vi "manejaBD.vi"(8 "error in":errorcluster, 10 "All Message Queues in":T1, 11 "Sonometro in":refnum<class "Sonometro.lvclass">) -> (0 "error out":errorcluster)   [LabVIEW 2019, in "Sonometro.lvclass"]
uses:
  Sonometro.lvclass
  QMH/Message Queue/All Message Queues.ctl
  QMH/Message Queue/Message Cluster.ctl
  Sonometro.lvclass/Sonometro.ctl
  <vilib>/Utility/error.llb/Error Cluster From Error Code.vi
  RerenceAllControlsToolkit/_get mutiple control reference by name.vi
  RerenceAllControlsToolkit/_get control reference by name.vi
  QMH/Message Queue/Enqueue Message (Single).vi
  <vilib>/ErrorRing/Error Ring.xnode
  Base de Datos/SQLiteConnector/SQLiteConnection.lvclass
  QMH/Message Queue/Message Queue.lvlib
  Base de Datos/Base de Datos.lvclass
  <vilib>/Utility/Data Type/NI_Data Type.lvlib
panel:
  out "All States":string[](array[string])
  out "Actual State":string
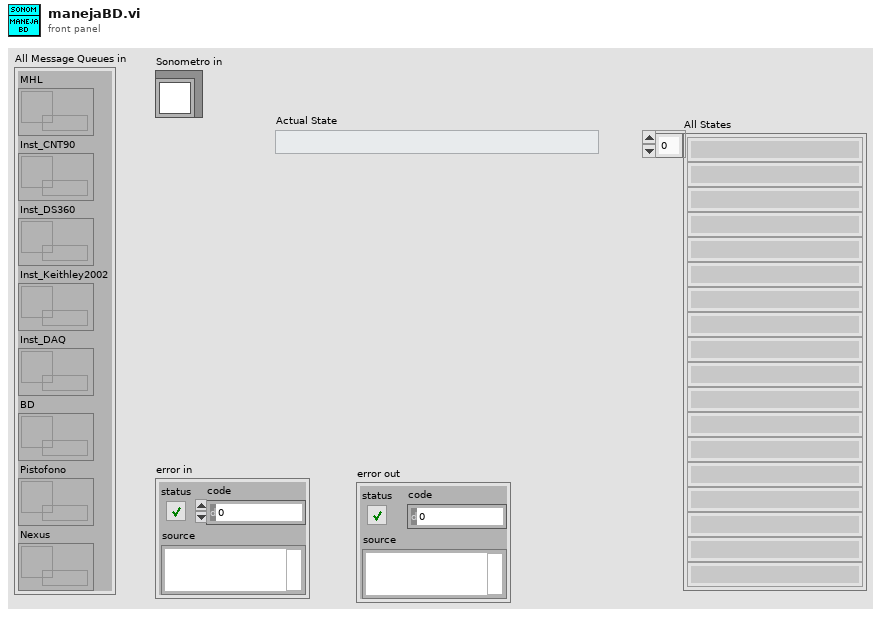
[diagram p1: front panel]
types:
  T1 = typedef "Message Queue.lvlib/All Message Queues.ctl" = cluster{"MHL":refnum<queue>, "Inst_CNT90":refnum<queue>, "Inst_DS360":refnum<queue>, "Inst_Keithley2002":refnum<queue>, "Inst_DAQ":refnum<queue>, "BD":refnum<queue>, "Pistofono":refnum<queue>, "Nexus":refnum<queue>}
  T2 = cluster{"Marca":string, "Referencia":cluster{"ControlName":string, "ControlReference":refnum<vi>}[]}
  T3 = typedef "NI_Data Type.lvlib/Data Type.ctl" = enum8{"Invalid Type", "Void", "I8", "I16", "I32", "I64", "U8", "U16", "U32", "U64", "Single Float", "Double Float", "Extended Float", "Single Complex", "Double Complex", "Extended Complex", "Enum U8", "Enum U16", "Enum U32", "Enum U64", "Single Float With Unit", "Double Float With Unit", "Extended Float With Unit", "Single Complex with Unit", "Double Complex with Unit", "Extended Complex with Unit", "Boolean", "String", "Path", "Picture", "Tag", "Array", "Cluster", "Variant", "LV Variant", "Waveform", "Timestamp", "Digital Waveform", "Digital Data", "ExpressData", "Refnum", "External Data", "VI", "Poly VI", "LabVIEW Class Instance", "Fixed Point", "Set Collection", "Map Collection"}
  T4 = cluster{"ControlName":string, "ControlReference":refnum<vi>}[]
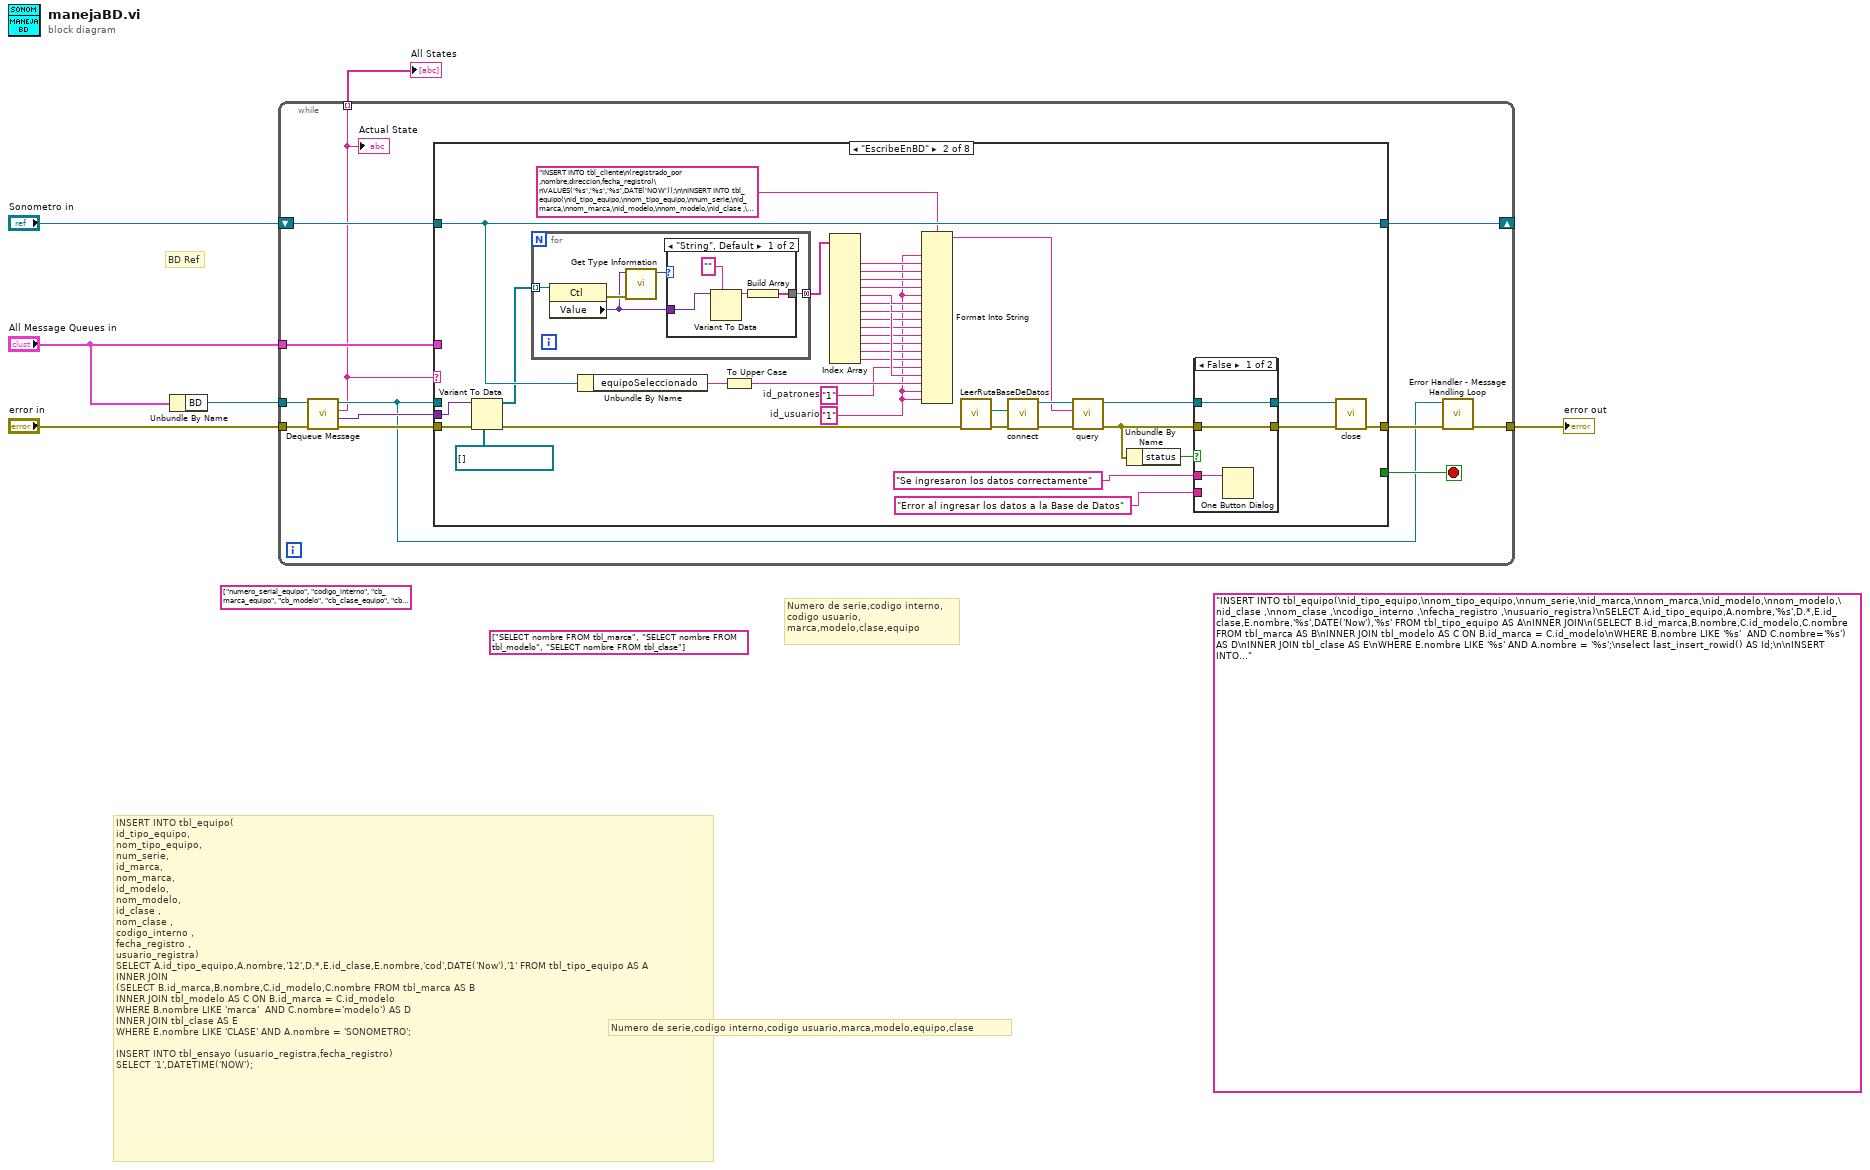
[diagram p0: block diagram]
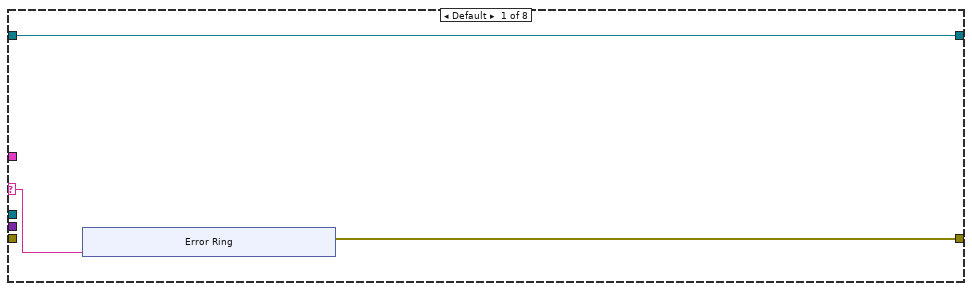
[diagram p2: hidden frame]
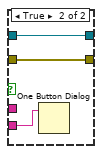
[diagram p3: hidden frame]
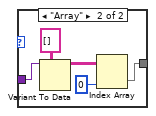
[diagram p4: hidden frame]
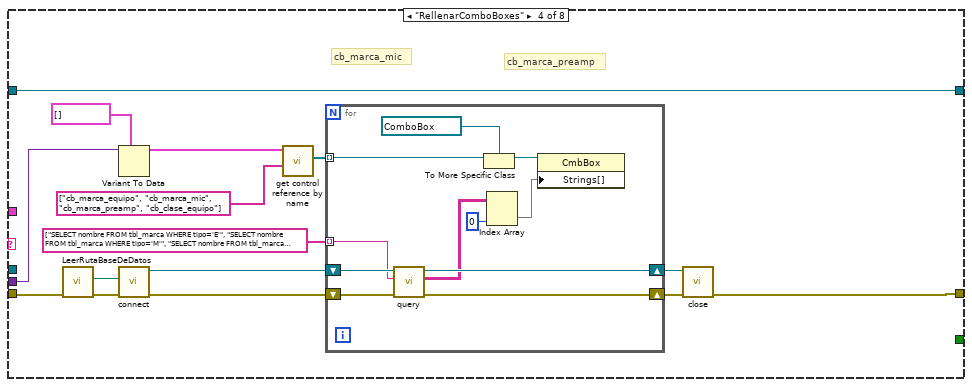
[diagram p6: hidden frame]
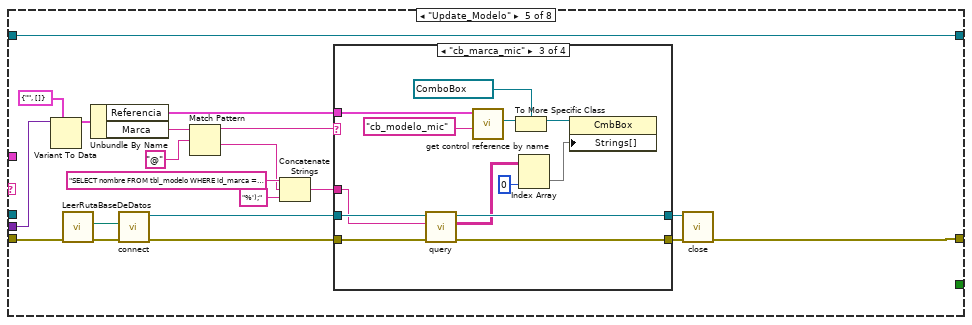
[diagram p7: hidden frame]
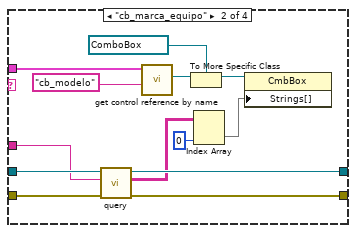
[diagram p9: hidden frame]
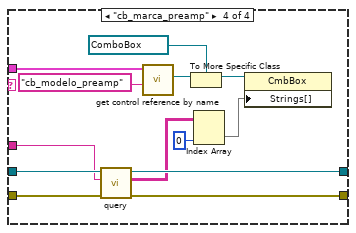
[diagram p10: hidden frame]
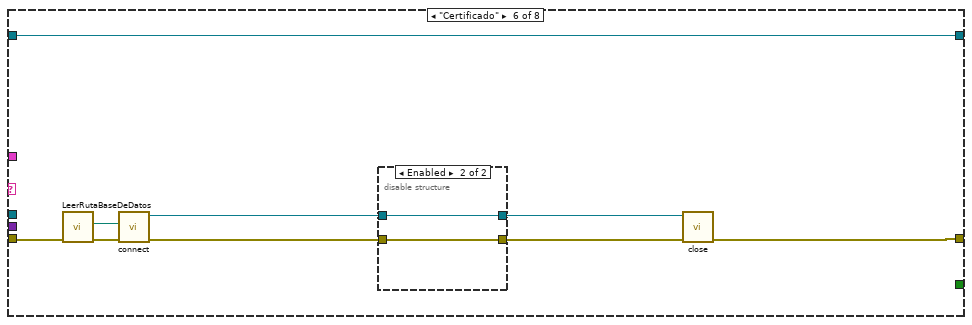
[diagram p11: hidden frame]
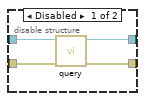
[diagram p12: hidden frame]
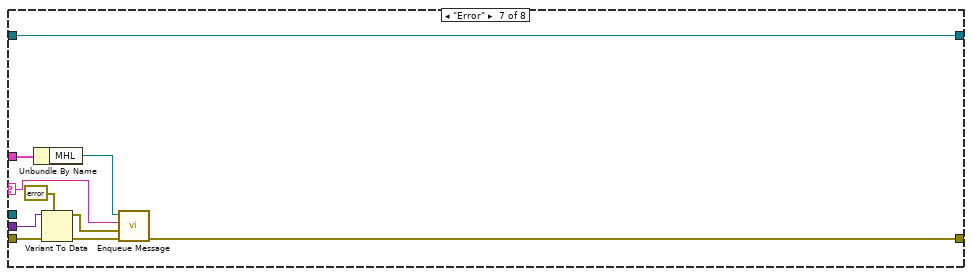
[diagram p13: hidden frame]
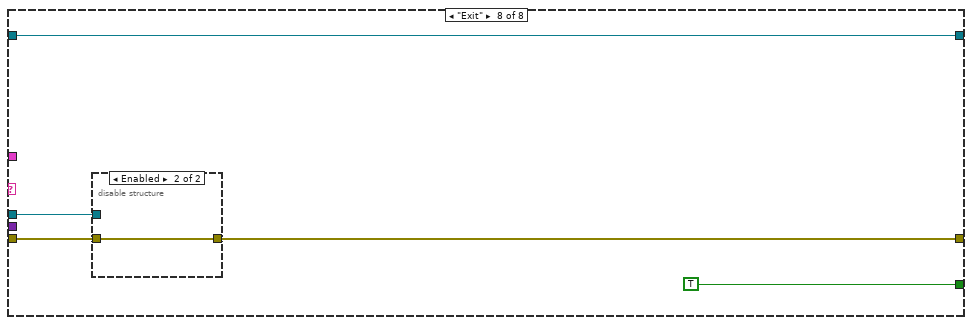
[diagram p14: hidden frame]
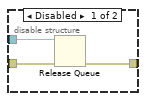
[diagram p15: hidden frame]
diagram:
  (unwired) string[] ["numero_serial_equipo", "codigo_interno", "cb_marca_equipo", "cb_modelo", "cb_clase_equipo", "cb_marca_mic", "cb_modelo_mic", "numero_serial_mic", "cb_marca_preamp", "cb_modelo_preamp", "numero_serial_preamp"]
  (unwired) "INSERT INTO tbl_equipo(\nid_tipo_equipo,\nnom_tipo_equipo,\nnum_serie,\nid_marca,\nnom_marca,\nid_modelo,\nnom_modelo,\nid_clase ,\nnom_clase ,\ncodigo_interno ,\nfecha_registro ,\nusuario_registra)\nSELECT A.id_tipo_equipo,A.nombre,'%s',D.*,E.id_clase,E.nombre,'%s',DATE('Now'),'%s' FROM tbl_tipo_equipo AS A\nINNER JOIN\n(SELECT B.id_marca,B.nombre,C.id_modelo,C.nombre FROM tbl_marca AS B\nINNER JOIN tbl_modelo AS C ON B.id_marca = C.id_modelo\nWHERE B.nombre LIKE '%s'  AND C.nombre='%s') AS D\nINNER JOIN tbl_clase AS E\nWHERE E.nombre LIKE '%s' AND A.nombre = '%s';\nselect last_insert_rowid() AS Id;\n\nINSERT INTO tbl_info_ensayo (id_ensayo,id_equipo,id_cliente,id_cond_amb_iniciales,id_clase_pruebas)\nSELECT (SELECT MAX(id_ensayo) FROM tbl_ensayo) AS id_ensayo,(SELECT MAX(id_equipo) FROM tbl_equipo) AS id_equipo,'%s' AS id_cliente,(SELECT MAX(id_cond_amb_iniciales) FROM tbl_cond_amb_iniciales) AS id_cond_amb_iniciales,\n(SELECT id_clase_prueba FROM tbl_clase_prueba WHERE id_clase=(SELECT id_clase FROM tbl_equipo ORDER BY id_equipo DESC LIMIT 1)  AND id_prueba=(SELECT id_prueba FROM tbl_prueba Where nombre='%s')) AS id_clase_pruebas;\n"
  (unwired) string[] ["SELECT nombre FROM tbl_marca", "SELECT nombre FROM tbl_modelo", "SELECT nombre FROM tbl_clase"]
  # "INSERT INTO tbl_equipo(\nid_tipo_equipo,\nnom_tipo_equipo,\nnum_serie,\nid_marca,\nnom_marca,\nid_modelo,\nnom_modelo,\nid_clase ,\nnom_clase ,\ncodigo_interno ,\nfecha_registro ,\nusuario_registra)\nSELECT A.id_tipo_equipo,A.nombre,'12',D.*,E.id_clase,E.nombre,'cod',DATE('Now'),'1' FROM tbl_tipo_equipo AS A\nINNER JOIN\n(SELECT B.id_marca,B.nombre,C.id_modelo,C.nombre FROM tbl_marca AS B\nINNER JOIN tbl_modelo AS C ON B.id_marca = C.id_modelo\nWHERE B.nombre LIKE 'marca'  AND C.nombre='modelo') AS D\nINNER JOIN tbl_clase AS E\nWHERE E.nombre LIKE 'CLASE' AND A.nombre = 'SONOMETRO';\n\nINSERT INTO tbl_ensayo (usuario_registra,fecha_registro)\nSELECT '1',DATETIME('NOW');"
  # "Numero de serie,codigo interno,\ncodigo usuario,\nmarca,modelo,clase,equipo"
  # "Numero de serie,codigo interno,codigo usuario,marca,modelo,equipo,clase"
  # "BD Ref"
  n1 = Unbundle By Name("All Message Queues in") -> ("BD"=w4:refnum<queue>)
  n2 = while {
    tunnel: "error in" -> [w18]
    tunnel: w4 -> [w17]
    tunnel: "All Message Queues in" -> [w16]
    tunnel: [w9] -> w2
    shift-right: [w12] -> _
    shift-left: "Sonometro in" -> [w15]
    tunnel: [w7] -> w1 mode=indexing
    stop <- w11 stop-if-true
    n3 = call "Dequeue Message.vi"("error in (no error)"=w18, "Message Queue"=w17) -> ("error out"=w13:errorcluster, "Message Data"=w14:variant, "Message"=w7:string, "dup Message Queue"=w8:refnum<queue>)  [unwired: 6 in]
    "Actual State" <- w7
    n4 = case shown="\"EscribeEnBD\"" w7 {
      selector: w7 -> [w21 _ _ _ _ _ w195 _]
      tunnel: w16 -> [_ _ _ _ _ _ w194 _]
      tunnel: w15 -> [w19 w61 w88 w89 w134 w184 w192 w202]
      tunnel: w8 -> [_ _ _ _ _ _ _ w204]
      tunnel: w14 -> [_ w63 _ w96 w126 _ w198 _]
      tunnel: w13 -> [_ w65 w87 w99 w129 w179 w199 w205]
      tunnel: [w20 w66 w87 w97 w127 w177 w191 w201] -> w10
      tunnel: [w19 w61 w88 w89 w134 w184 w192 w202] -> w12
      tunnel: [_ _ _ _ _ _ _ TRUE] -> w11
      frame Default {
        n5 = xnode "Error Ring"("parameter 0"=w21) -> ("error out"=w20:errorcluster)
      }
      frame "EscribeEnBD" {
        w47 = "1"  # id_patrones
        w36 = "1"  # id_usuario
        n6 = Variant To Data(error in=w65, type=refnum<vi>[] [], Variant=w63) -> (data=w40:refnum<vi>[], error out=w64:errorcluster)
        n7 = for {
          tunnel: w40 -> [w77] mode=indexing
          tunnel: [w76] -> w39 mode=concatenating
          n8 = property class="Ctl"(reference=w77) -> (error out=w75:errorcluster, "Value"=w74:variant)  [unwired: 1 in, 1 out]
          n9 = call <vilib>:"Get Type Information.vi"("error in (no error)"=w75, "variant"=w74) -> ("type"=w73:T3)  [unwired: 5 in, 4 out]
          n10 = case shown="\"String\", Default" w73 {
            tunnel: [w78 w83] -> w76
            tunnel: w74 -> [w80 w85]
            frame "String", Default {
              n11 = Variant To Data(type="", Variant=w80) -> (data=w79:string)  [unwired: 1 in, 1 out]
              n12 = Build Array(w79) -> (w78:string[])
            }
            frame "Array" {
              n13 = Variant To Data(type=string[][] [], Variant=w85) -> (data=w84:string[][])  [unwired: 1 in, 1 out]
              n14 = Index Array(array=w84, index (col)=0 ("disabled index (col)")) -> (element=w83:string[])  [unwired: 1 in]
            }
          }
        }
        n15 = Unbundle By Name(w61) -> ("equipoSeleccionado"=w50:string)
        n16 = To Upper Case(1:w50) -> (0:w49:string)
        n17 = Index Array(array=w39) -> (element #2=w37:string, element #3=w38:string, element #4=w55:string, element #5=w54:string, element #6=w53:string, element #7=w52:string, element #8=w48:string, element #9=w46:string, element #10=w45:string, element #11=w44:string, element #12=w43:string, element #13=w42:string, element #14=w41:string)  [unwired: 14 in, 1 out]
        n18 = Format Into String(format string="INSERT INTO tbl_cliente\n(registrado_por ,nombre,direccion,fecha_registro)\nVALUES('%s','%s','%s',DATE('NOW'));\n\nINSERT INTO tbl_equipo(\nid_tipo_equipo,\nnom_tipo_equipo,\nnum_serie,\nid_marca,\nnom_marca,\nid_modelo,\nnom_modelo,\nid_clase ,\nnom_clase ,\ncodigo_interno ,\nfecha_registro ,\nusuario_registra,\nmarca_microfono,\nmodelo_microfono,\nnum_serie_microfono,\nmarca_preamplificador ,\nmodelo_preamplificador,\nnum_serie_preamplificador,\nid_patrones_calib)\nSELECT A.id_tipo_equipo,A.nombre,'%s',D.*,E.id_clase,E.nombre,'%s',DATE('Now'),'%s',F.* FROM tbl_tipo_equipo AS A\nINNER JOIN\n(SELECT B.id_marca,B.nombre,C.id_modelo,C.nombre FROM tbl_marca AS B\nINNER JOIN tbl_modelo AS C ON B.id_marca = C.id_marca\nWHERE B.nombre LIKE '%s'  AND C.nombre='%s') AS D\nINNER JOIN tbl_clase AS E\nINNER JOIN (SELECT '%s','%s','%s','%s','%s','%s','%s') AS F\nWHERE E.nombre LIKE '%s' AND A.nombre = '%s';\n\nINSERT INTO tbl_equipo_cliente(id_cliente,nom_cliente,id_equipo,fecha_registro,usuario_registra)\nSELECT MAX(id_cliente),nombre,last_insert_rowid(),DATETIME('NOW'),'%s' FROM tbl_cliente;\n\nINSERT INTO tbl_ensayo (usuario_registra,fecha_registro)\nSELECT '%s',DATETIME('NOW');\n", w36, w37, w38, w55, w54, w36, w53, w52, w46, w45, w44, w43, w42, w41, w47, w48, w49, w36, w36) -> (resulting string=w51:string)  [unwired: 2 in, 1 out]
        n19 = call "LeerRutaBaseDeDatos.vi"("error in (no error)"=w64) -> ("error out"=w58:errorcluster, "Database Path"=w57:path)  [unwired: 9 in]
        n20 = call "connect.vi"("error in (no error)"=w58, "Database Path"=w57) -> ("error out"=w60:errorcluster, "object out"=w59:refnum<class "SQLiteConnection.lvclass">)  [unwired: 8 in]
        n21 = call "query.vi"("error in (no error)"=w60, "SQL Statement"=w51, "object in"=w59) -> ("error out"=w32:errorcluster, "object out"=w34:refnum<class "SQLiteConnection.lvclass">)  [unwired: 5 in, 2 out]
        n22 = Unbundle By Name(w32) -> ("status"=w35:bool)
        n23 = case shown="False" w35 {
          tunnel: w34 -> [w69 w72]
          tunnel: [w69 w72] -> w33
          tunnel: w32 -> [w68 w71]
          tunnel: [w68 w71] -> w31
          tunnel: "Se ingresaron los datos correctamente" -> [w67 _]
          tunnel: "Error al ingresar los datos a la Base de Datos" -> [_ w70]
          frame False {
            n24 = One Button Dialog(message=w67) -> ()  [unwired: 1 in, 1 out]
          }
          frame True {
            n25 = One Button Dialog(message=w70) -> ()  [unwired: 1 in, 1 out]
          }
        }
        n26 = call-dynamic "close.vi"("error in (no error)"=w31, "object in"=w33) -> ("error out"=w66:errorcluster)  [unwired: 8 in, 1 out]
      }
      frame "Initialize" {
      }
      frame "RellenarComboBoxes" {
        # "cb_marca_preamp"
        # "cb_marca_mic"
        n27 = call "LeerRutaBaseDeDatos.vi"("error in (no error)"=w99) -> ("error out"=w101:errorcluster, "Database Path"=w100:path)  [unwired: 9 in]
        n28 = Variant To Data(type=cluster{string, refnum<vi>}[] [] ("Control references"), Variant=w96) -> (data=w94:cluster{string, refnum<vi>}[])  [unwired: 1 in, 1 out]
        n29 = call "connect.vi"("error in (no error)"=w101, "Database Path"=w100) -> ("error out"=w102:errorcluster, "object out"=w103:refnum<class "SQLiteConnection.lvclass">)  [unwired: 8 in]
        n30 = call-poly "get control reference by name.vi"("Control names"=string[] ["cb_marca_equipo", "cb_marca_mic", "cb_marca_preamp", "cb_clase_equipo"] ("Control name"), "Control references"=w94) -> ("References"=w92:refnum<vi>[])  [unwired: 4 in, 1 out]
        n31 = for {
          tunnel: w92 -> [w109] mode=indexing
          shift-right: [w112] -> w98
          shift-left: w103 -> [w114]
          shift-right: [w105] -> w91
          shift-left: w102 -> [w113]
          tunnel: string[] ["SELECT nombre FROM tbl_marca WHERE tipo='E'", "SELECT nombre FROM tbl_marca WHERE tipo='M'", "SELECT nombre FROM tbl_marca WHERE tipo='P'", "SELECT nombre FROM tbl_clase"] -> [w104] mode=indexing
          n32 = call "query.vi"("error in (no error)"=w113, "SQL Statement"=w104, "object in"=w114) -> ("error out"=w105:errorcluster, "result"=w111:string[][], "object out"=w112:refnum<class "SQLiteConnection.lvclass">)  [unwired: 5 in, 1 out]
          n33 = To More Specific Class(target class=refnum<vi> refnum ("cb_marca_equipo"), reference=w109) -> (specific class reference=w108:refnum<vi>)  [unwired: 1 in, 1 out]
          n34 = Index Array(array=w111, index (col)=0 ("disabled index (col)")) -> (element=w106:string[])  [unwired: 1 in]
          n35 = property class="CmbBox"(reference=w108, "Strings[]"=w106) -> ()  [unwired: 1 in, 2 out]
        }
        n36 = call-dynamic "close.vi"("error in (no error)"=w91, "object in"=w98) -> ("error out"=w97:errorcluster)  [unwired: 8 in, 1 out]
      }
      frame "Update_Modelo" {
        n37 = Variant To Data(type=T2 {"Marca"="", "Referencia"=[]} ("output cluster"), Variant=w126) -> (data=w123:T2)  [unwired: 1 in, 1 out]
        n38 = call "LeerRutaBaseDeDatos.vi"("error in (no error)"=w129) -> ("error out"=w131:errorcluster, "Database Path"=w130:path)  [unwired: 9 in]
        n39 = Unbundle By Name(w123) -> ("Referencia"=w122:T4, "Marca"=w120:string)
        n40 = call "connect.vi"("error in (no error)"=w131, "Database Path"=w130) -> ("error out"=w132:errorcluster, "object out"=w133:refnum<class "SQLiteConnection.lvclass">)  [unwired: 8 in]
        n41 = Match Pattern(string=w120, regular expression="@") -> (before substring=w121:string, after substring=w117:string)  [unwired: 1 in, 2 out]
        n42 = Concatenate Strings("SELECT nombre FROM tbl_modelo WHERE id_marca = (SELECT id_marca FROM tbl_marca WHERE nombre LIKE '%" ("SQL Statement"), w117, "%');" ("string")) -> (w115:string)
        n43 = case shown="\"cb_marca_mic\"" w121 {
          tunnel: w133 -> [w136 w149 w162 w175]
          tunnel: w132 -> [w135 w148 w161 w174]
          tunnel: [w136 w147 w160 w173] -> w128
          tunnel: [w135 w145 w158 w171] -> w125
          tunnel: w122 -> [_ w138 w151 w164]
          tunnel: w115 -> [_ w137 w150 w163]
          frame "False", Default {
          }
          frame "cb_marca_equipo" {
            n44 = call "query.vi"("error in (no error)"=w148, "SQL Statement"=w137, "object in"=w149) -> ("error out"=w145:errorcluster, "result"=w144:string[][], "object out"=w147:refnum<class "SQLiteConnection.lvclass">)  [unwired: 5 in, 1 out]
            n45 = call-poly "get control reference by name.vi"("Control name"="cb_modelo", "Control references"=w138) -> ("Ctl Refnum"=w146:refnum<vi>)  [unwired: 4 in, 1 out]
            n46 = To More Specific Class(target class=refnum<vi> refnum ("cb_marca_equipo"), reference=w146) -> (specific class reference=w142:refnum<vi>)  [unwired: 1 in, 1 out]
            n47 = Index Array(array=w144, index (col)=0 ("disabled index (col)")) -> (element=w140:string[])  [unwired: 1 in]
            n48 = property class="CmbBox"(reference=w142, "Strings[]"=w140) -> ()  [unwired: 1 in, 2 out]
          }
          frame "cb_marca_mic" {
            n49 = call "query.vi"("error in (no error)"=w161, "SQL Statement"=w150, "object in"=w162) -> ("error out"=w158:errorcluster, "result"=w157:string[][], "object out"=w160:refnum<class "SQLiteConnection.lvclass">)  [unwired: 5 in, 1 out]
            n50 = call-poly "get control reference by name.vi"("Control name"="cb_modelo_mic", "Control references"=w151) -> ("Ctl Refnum"=w159:refnum<vi>)  [unwired: 4 in, 1 out]
            n51 = To More Specific Class(target class=refnum<vi> refnum ("cb_marca_equipo"), reference=w159) -> (specific class reference=w155:refnum<vi>)  [unwired: 1 in, 1 out]
            n52 = Index Array(array=w157, index (col)=0 ("disabled index (col)")) -> (element=w153:string[])  [unwired: 1 in]
            n53 = property class="CmbBox"(reference=w155, "Strings[]"=w153) -> ()  [unwired: 1 in, 2 out]
          }
          frame "cb_marca_preamp" {
            n54 = call "query.vi"("error in (no error)"=w174, "SQL Statement"=w163, "object in"=w175) -> ("error out"=w171:errorcluster, "result"=w170:string[][], "object out"=w173:refnum<class "SQLiteConnection.lvclass">)  [unwired: 5 in, 1 out]
            n55 = call-poly "get control reference by name.vi"("Control name"="cb_modelo_preamp", "Control references"=w164) -> ("Ctl Refnum"=w172:refnum<vi>)  [unwired: 4 in, 1 out]
            n56 = To More Specific Class(target class=refnum<vi> refnum ("cb_marca_equipo"), reference=w172) -> (specific class reference=w168:refnum<vi>)  [unwired: 1 in, 1 out]
            n57 = Index Array(array=w170, index (col)=0 ("disabled index (col)")) -> (element=w166:string[])  [unwired: 1 in]
            n58 = property class="CmbBox"(reference=w168, "Strings[]"=w166) -> ()  [unwired: 1 in, 2 out]
          }
        }
        n59 = call-dynamic "close.vi"("error in (no error)"=w125, "object in"=w128) -> ("error out"=w127:errorcluster)  [unwired: 8 in, 1 out]
      }
      frame "Certificado" {
        n60 = call "LeerRutaBaseDeDatos.vi"("error in (no error)"=w179) -> ("error out"=w181:errorcluster, "Database Path"=w180:path)  [unwired: 9 in]
        n61 = call "connect.vi"("error in (no error)"=w181, "Database Path"=w180) -> ("error out"=w182:errorcluster, "object out"=w183:refnum<class "SQLiteConnection.lvclass">)  [unwired: 8 in]
        n62 = disable-structure shown="Enabled" {
          disable-tunnel: w183 -> [w188 w190]
          disable-tunnel: w182 -> [w187 w189]
          disable-tunnel: [w186 w190] -> w178
          disable-tunnel: [w185 w189] -> w176
          frame Disabled {
            n63 = call "query.vi"("error in (no error)"=w187, "object in"=w188) -> ("error out"=w185:errorcluster, "object out"=w186:refnum<class "SQLiteConnection.lvclass">)  [unwired: 6 in, 2 out]
          }
          frame Enabled {
          }
        }
        n64 = call-dynamic "close.vi"("error in (no error)"=w176, "object in"=w178) -> ("error out"=w177:errorcluster)  [unwired: 8 in, 1 out]
      }
      frame "Error" {
        n65 = Unbundle By Name(w194) -> ("MHL"=w193:refnum<queue>)
        n66 = Variant To Data(error in=w199, type=errorcluster {"status"=FALSE, "code"=0, "source"=""} ("error constant"), Variant=w198) -> (data=w196:errorcluster, error out=w197:errorcluster)
        n67 = call-poly "Enqueue Message.vi"("error in (no error)"=w197, "Message Data"=w196, "Message"=w195, "Message Queue"=w193) -> ("error out"=w191:errorcluster)  [unwired: 6 in, 1 out]
      }
      frame "Exit" {
        n68 = disable-structure shown="Enabled" {
          disable-tunnel: w205 -> [w208 w209]
          disable-tunnel: w204 -> [w207 _]
          disable-tunnel: [w206 w209] -> w201
          frame Disabled {
            n69 = Release Queue(queue=w207, error in (no error)=w208) -> (error out=w206:errorcluster)  [unwired: 1 in, 2 out]
          }
          frame Enabled {
          }
        }
      }
    }
    n70 = call "Error Handler - Message Handling Loop.vi"("error in (no error)"=w10, "Message Queue"=w8) -> ("dup error in"=w9:errorcluster)  [unwired: 8 in, 1 out]
  }
  "error out" <- w2
  "All States" <- w1
